vi "Remove Points too Close Togther.vi"(7 "Distance Threshold":dbl=2.9, 10 "Columns":i32[](array[numeric]), 11 "Rows":i32[](array[numeric])) -> (2 "Columns Out":i32[](array[numeric]), 3 "Rows Out":i32[](array[numeric]))   [LabVIEW 2017, in "AntFarm_MB.lvclass"]
uses:
  AntFarm_MB.lvclass
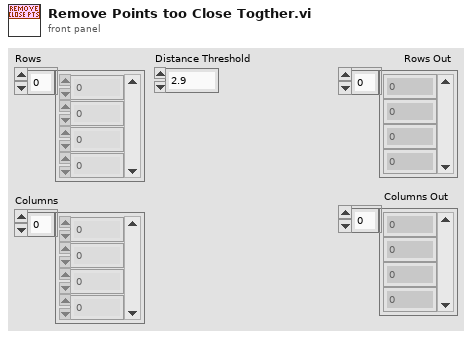
[diagram p1: front panel]
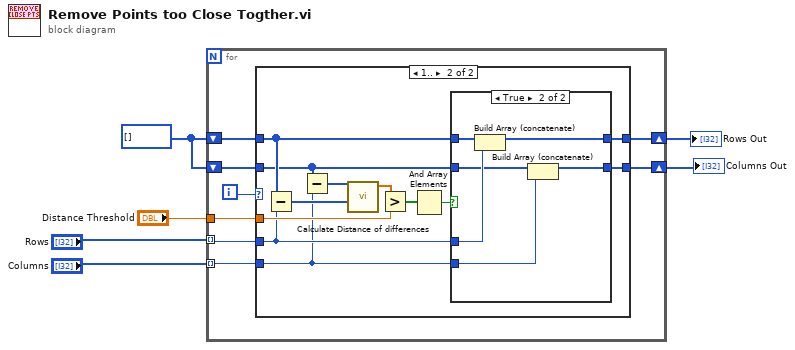
[diagram p0: block diagram]
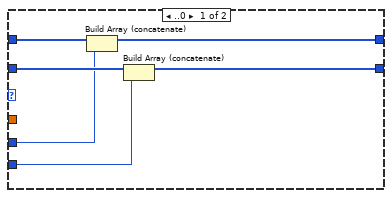
[diagram p2: hidden frame]
diagram:
  w3 = i32[] [] ("Danger Rows Out 3")
  n1 = for {
    tunnel: "Rows" -> [w11] mode=indexing
    tunnel: "Columns" -> [w10] mode=indexing
    shift-right: [w8] -> w5
    shift-left: w3 -> [w13]
    shift-right: [w9] -> w6
    shift-left: w3 -> [w12]
    tunnel: "Distance Threshold" -> [w14]
    i -> [w7]
    n2 = case shown="1.." w7 {
      tunnel: w14 -> [_ w29]
      tunnel: w13 -> [w20 w26]
      tunnel: w12 -> [w18 w25]
      tunnel: w11 -> [w16 w24]
      tunnel: w10 -> [w15 w23]
      tunnel: [w17 w22] -> w9
      tunnel: [w19 w21] -> w8
      frame ..0 {
        n3 = Build Array (concatenate)(w20, w16) -> (w19:i32[])
        n4 = Build Array (concatenate)(w18, w15) -> (w17:i32[])
      }
      frame 1.. {
        n5 = Subtract(x=w26, y=w24) -> (x-y=w31:i32[])
        n6 = Subtract(x=w25, y=w23) -> (x-y=w32:i32[])
        n7 = call "Calculate Distance of differences.vi"("Column Differences"=w31, "Row Differences"=w32) -> ("Array 3"=w30:dbl[])  [unwired: 9 in]
        n8 = Greater?(x=w30, y=w29) -> (0:w28:bool[])
        n9 = And Array Elements(Boolean array=w28) -> (logical AND=w27:bool)
        n10 = case shown="True" w27 {
          tunnel: w26 -> [w34 w40]
          tunnel: w25 -> [w33 w38]
          tunnel: w24 -> [_ w39]
          tunnel: w23 -> [_ w35]
          tunnel: [w33 w37] -> w22
          tunnel: [w34 w36] -> w21
          frame False {
          }
          frame True {
            n11 = Build Array (concatenate)(w40, w39) -> (w36:i32[])
            n12 = Build Array (concatenate)(w38, w35) -> (w37:i32[])
          }
        }
      }
    }
  }
  "Columns Out" <- w6
  "Rows Out" <- w5
